vi "Read Channel Settings ID.vi"(8 "error in (no error)":errorcluster, 10 "Channel ID":string, 11 "Configuration Session in":refnum<class "Configuration Session.lvclass">) -> (0 "error out":errorcluster, 1 "Settings ID":string, 3 "Configuration Session out":refnum<class "Configuration Session.lvclass">, 4 "found?":bool)   [LabVIEW 2017, in "DSF Configuration.lvlib" / "Configuration Session.lvclass"]
uses:
  Configuration Session.lvclass
  Configuration Session.lvclass/Configuration Session.ctl
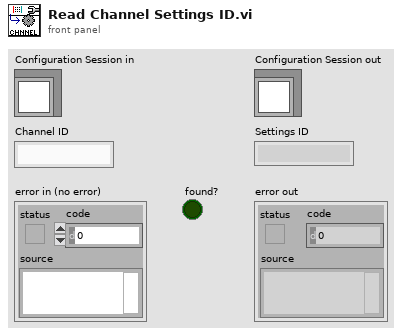
[diagram p1: front panel]
types:
  T1 = typedef "DSF Configuration.lvlib/Configuration Session.lvclass/DSF Config Data Ref.ctl" = refnum<data-value>
  T2 = typedef "DSF Configuration.lvlib/Configuration Session.lvclass/DSF Config Data.ctl" = cluster{"dsf configuration":T3, "path":path, "dirty":bool}
  T3 = typedef "DSF Configuration.lvlib/Configuration Session.lvclass/Internal.DSF Configuration.ctl" = cluster{"dsfversion":T4, "version":T4, "plugins":T5[], "groups":T8[], "transfers":T10[], "channels":T12[], "settings":T14[]}
  T4 = typedef "DSF Configuration.lvlib/DSF Version Info.ctl" = cluster{"major":u32, "minor":u32, "fix":u32, "build":string}
  T5 = typedef "DSF Configuration.lvlib/Configuration Session.lvclass/Internal.DSF Plugin with ID.ctl" = cluster{"id":string, "values":T6}
  T6 = typedef "DSF Configuration.lvlib/Configuration Session.lvclass/Internal.DSF Plugin Info.ctl" = cluster{"type":string, "timing":T7, "group ids":string[], "settings id":string}
  T7 = typedef "DSF Configuration.lvlib/DSF Timing Info.ctl" = cluster{"priority":u64, "decimation":u64, "offset":u64}
  T8 = typedef "DSF Configuration.lvlib/Configuration Session.lvclass/Internal.DSF Group with ID.ctl" = cluster{"id":string, "values":T9}
  T9 = typedef "DSF Configuration.lvlib/Configuration Session.lvclass/Internal.DSF Group Info.ctl" = cluster{"direction":i32, "timing":T7, "transfer ids":string[], "settings id":string}
  T10 = typedef "DSF Configuration.lvlib/Configuration Session.lvclass/Internal.DSF Transfer with ID.ctl" = cluster{"id":string, "values":T11}
  T11 = typedef "DSF Configuration.lvlib/Configuration Session.lvclass/Internal.DSF Transfer Info.ctl" = cluster{"byte order":i32, "channel ids":string[], "settings id":string}
  T12 = typedef "DSF Configuration.lvlib/Configuration Session.lvclass/Internal.DSF Channel with ID.ctl" = cluster{"id":string, "values":T13}
  T13 = typedef "DSF Configuration.lvlib/Configuration Session.lvclass/Internal.DSF Channel Info.ctl" = cluster{"count":u64, "buffer offset":u64, "data type":i32, "settings id":string}
  T14 = typedef "DSF Configuration.lvlib/Configuration Session.lvclass/Internal.DSF Settings with ID.ctl" = cluster{"id":string, "values":T15}
  T15 = typedef "DSF Configuration.lvlib/Configuration Session.lvclass/Internal.DSF Settings Info.ctl" = cluster{"key":string, "value":string}[]
  T16 = typedef "DSF Configuration.lvlib/DSF Group Info.ctl" = cluster{"direction":T17, "timing":T7, "transfer ids":string[], "settings id":string}
  T17 = typedef "DSF Configuration.lvlib/DSF Direction.ctl" = enum8{"Tx", "Rx"}
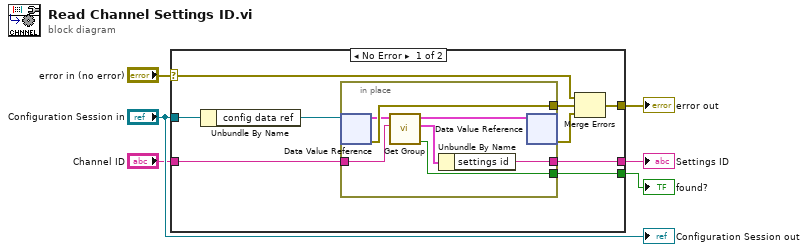
[diagram p0: block diagram]
diagram:
  n1 = case shown="No Error" "error in (no error)" {
    selector: "error in (no error)" -> [w15 w23]
    tunnel: "Configuration Session in" -> [w8 _]
    tunnel: [w13 w23] -> w4
    tunnel: "Channel ID" -> [w14 _]
    tunnel: [w10 _] -> w2
    tunnel: [w9 _] -> w1
    frame No Error {
      n2 = Unbundle By Name(w8) -> ("config data ref"=w7:T1)
      n3 = in-place {
        in-place-border: w14 -> [w20]
        in-place-border: [w22] -> w12
        in-place-border: [w19] -> w10
        in-place-border: [w16] -> w9
        n4 = in-place-dvr #1(w7) -> (w21:T2, w22:errorcluster)
        n5 = call "Get Group.vi"("id"=w20, "DSF Configuration in"=w21) -> ("exists?"=w19:bool, "info"=w17:T16, "DSF Configuration out"=w18:T2)  [unwired: 6 in, 1 out]
        n6 = Unbundle By Name(w17) -> ("settings id"=w16:string)
        n7 = in-place-dvr #1(w18) -> (w11:errorcluster)  [unwired: 1 out]
      }
      n8 = Merge Errors(w15, w12, w11) -> (w13:errorcluster)
    }
    frame Error {
    }
  }
  "error out" <- w4
  "found?" <- w2
  "Settings ID" <- w1
  "Configuration Session out" <- "Configuration Session in"
